vi "relu.vi"(1 "Array":dbl[](array[numeric])) -> (0 ">=0":dbl[](array[numeric]))   [LabVIEW 2023]
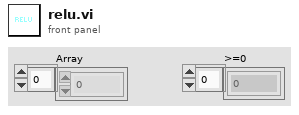
[diagram p1: front panel]
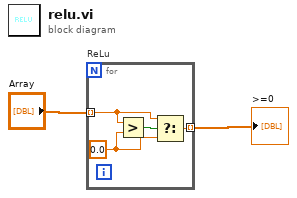
[diagram p0: block diagram]
diagram:
  n1 = for "ReLu" {
    tunnel: "Array" -> [w4] mode=indexing
    tunnel: [w3] -> w2 mode=indexing
    w5 = 0.0 ("f")
    n2 = Greater?(x=w4, y=w5) -> (0:w6:bool)
    n3 = Select(t=w4, s=w6, f=w5) -> (s? t:f=w3:dbl)
  }
  ">=0" <- w2
